vi "Script Tester.vi"() -> ()   [LabVIEW 2014]
panel:
  out "IN":bool
  out "OUT":bool
  in  "Execution Speed":u32(slide) scale=0.0..2000.0
  out "Function Code":picture
  out "Function Icon":picture
  in  "Evaluate":bool
  in  "OK":bool
  out "Status Msg":string
  out "Script":string
  in  "Test Script Path":path
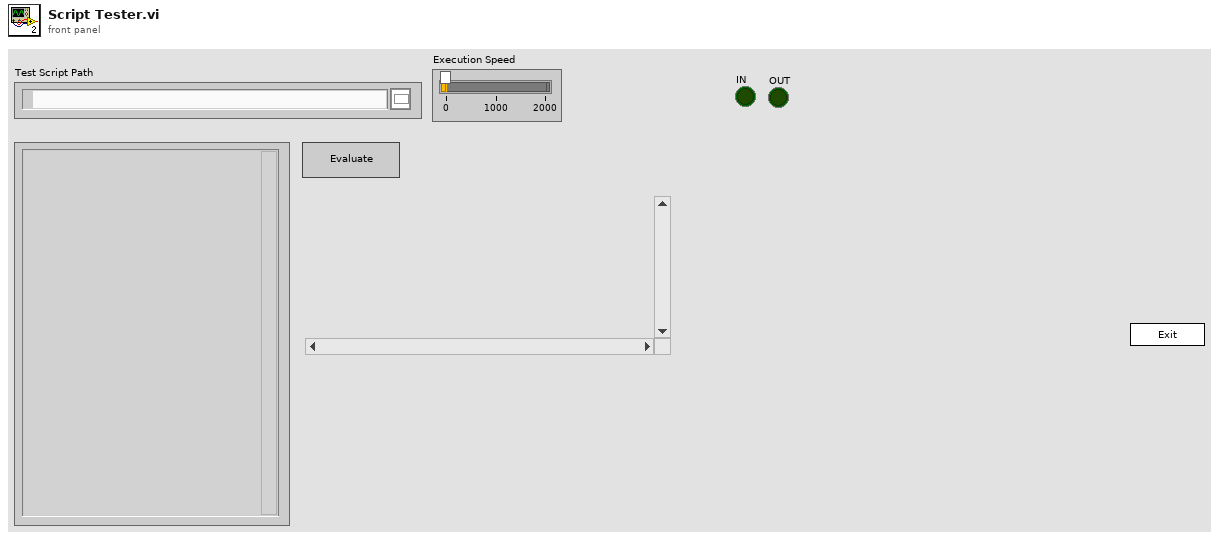
[diagram p1: front panel]
types:
  T1 = enum32{"invalid app kind", "Development System", "Run Time System", "Student Edition", "Embedded LabVIEW", "Evaluation", "Custom"}
  T2 = enum32{"Invalid", "Standard", "Closed", "Hidden", "Minimized", "Maximized"}
  T3 = enum32{"Bad", "Idle", "Run top level", "Running"}
  T4 = cluster{"Core":cluster{"Current VI Reference":refnum<vi>, "Close Panel on Exit?":bool}, "Test Script Path":path, "Script":string, "Function Path":path, "Script Pins":string[], "Function Pins":string[], "Function VI Ref":refnum<vi>}
  T5 = cluster{"Current VI Reference":refnum<vi>, "Close Panel on Exit?":bool}
  T6 = typedef "imagedata.ctl" = cluster{"image type":i32, "image depth":i32, "image":u8[], "mask":u8[], "colors":u32[], "Rectangle":cluster{"left":i16, "top":i16, "right":i16, "bottom":i16}}
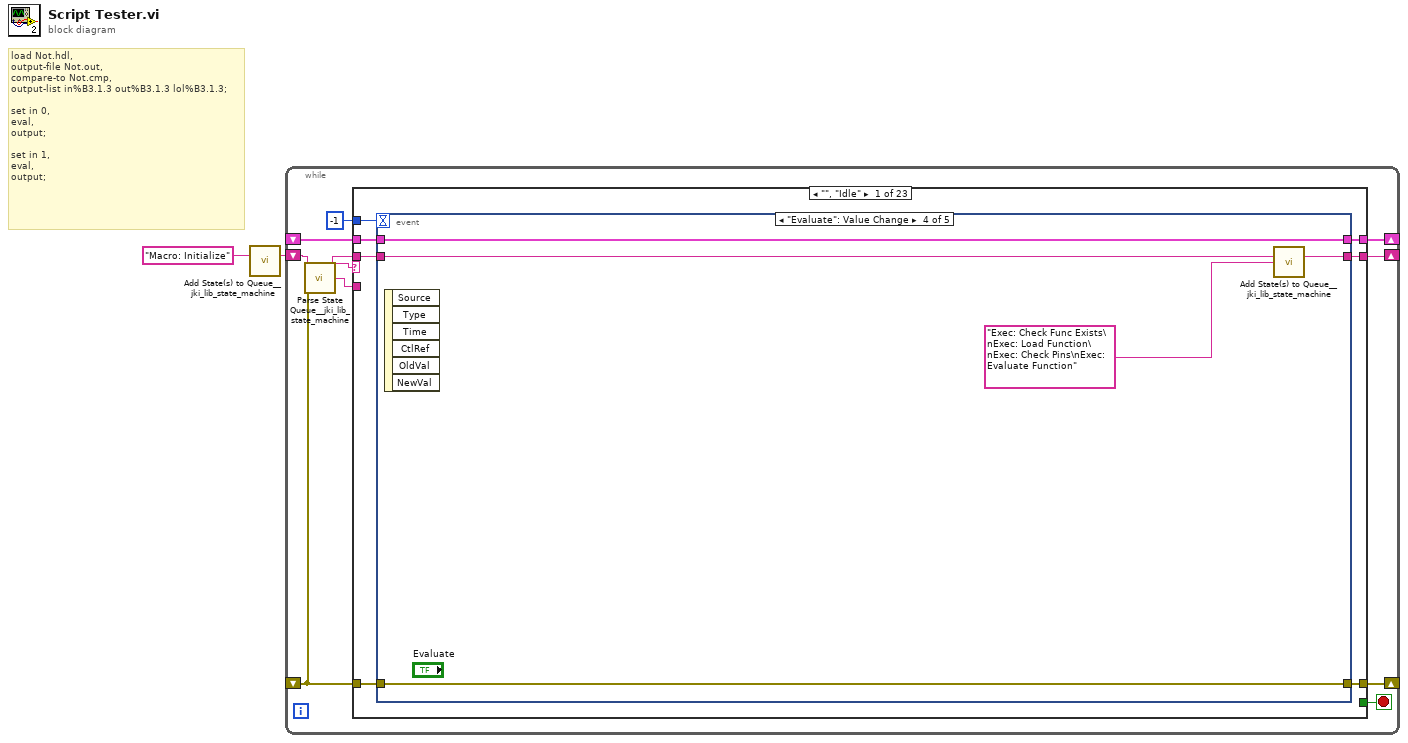
[diagram p0: block diagram]
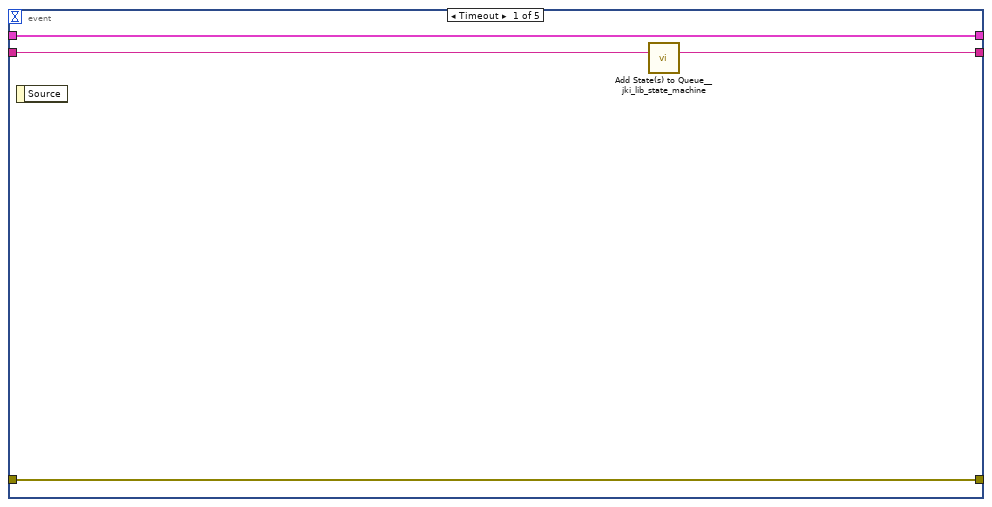
[diagram p2: hidden frame]
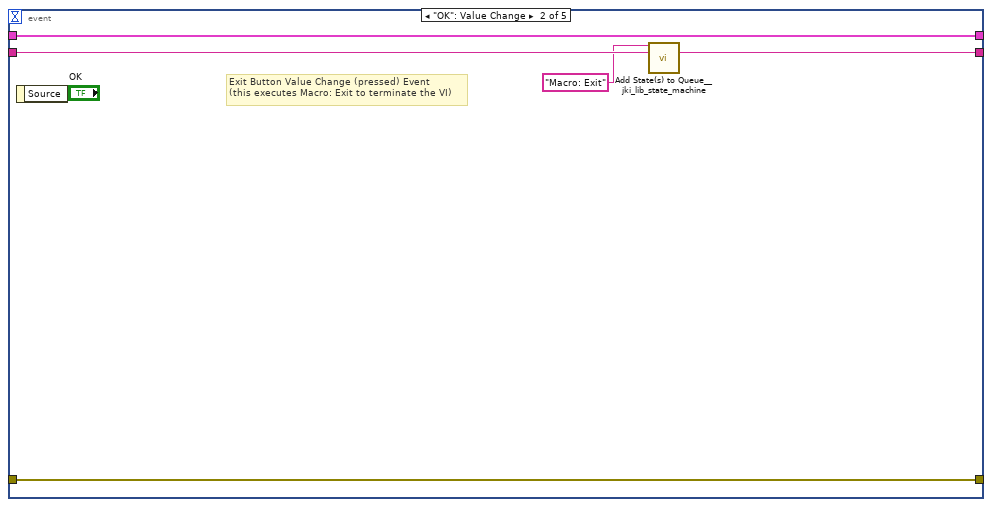
[diagram p3: hidden frame]
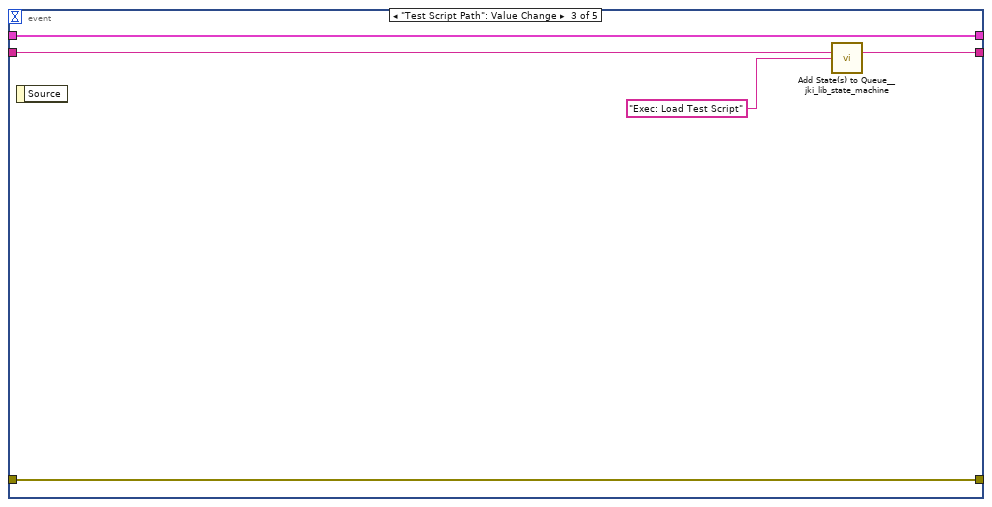
[diagram p4: hidden frame]
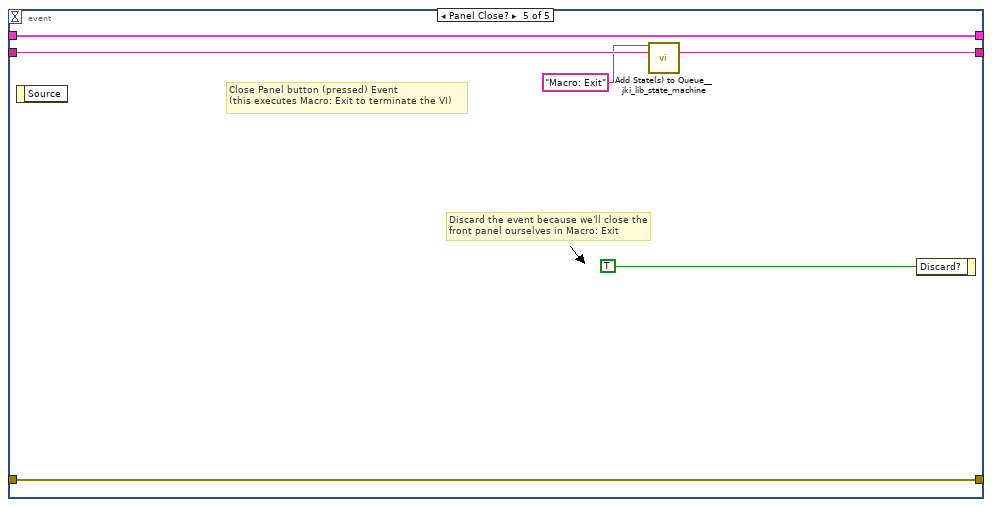
[diagram p5: hidden frame]
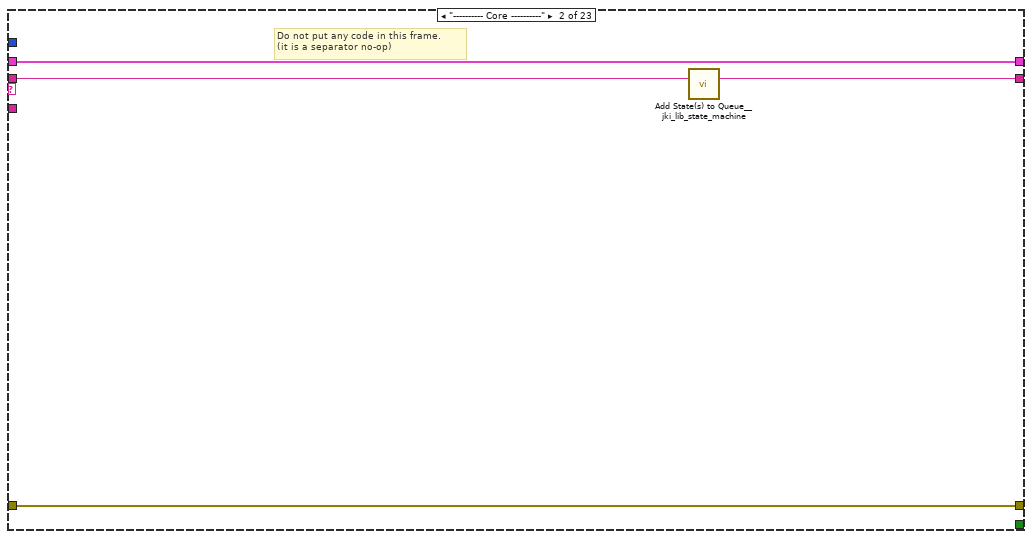
[diagram p6: hidden frame]
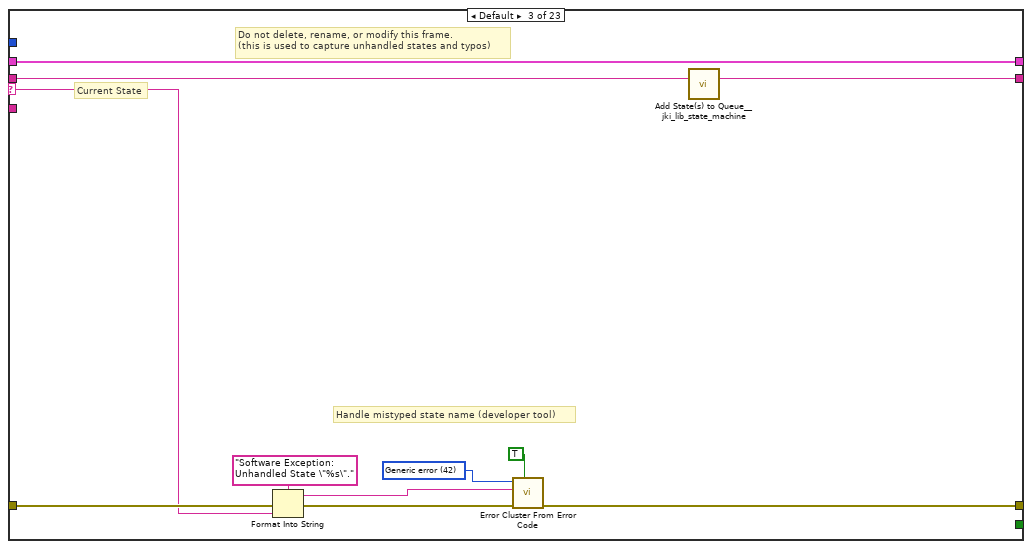
[diagram p7: hidden frame]
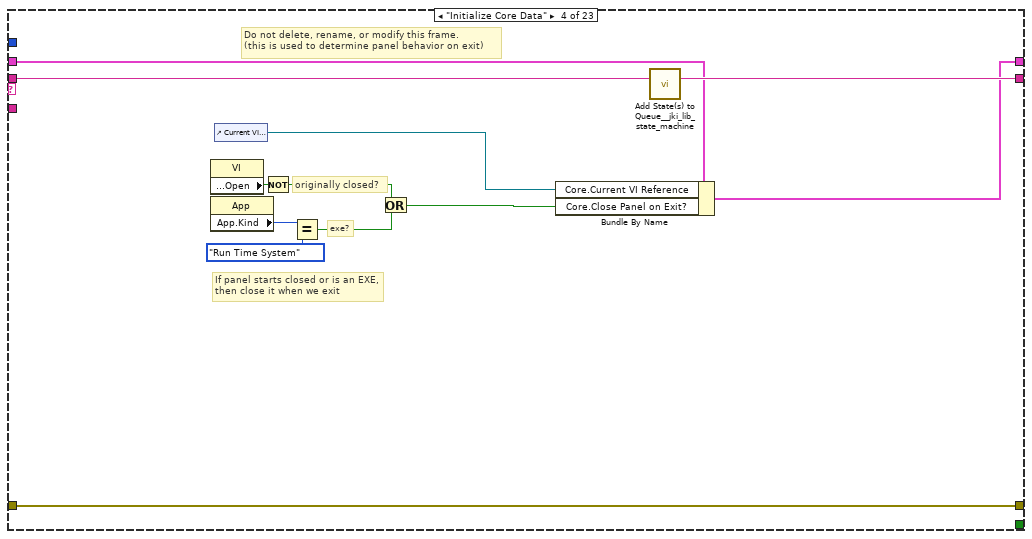
[diagram p8: hidden frame]
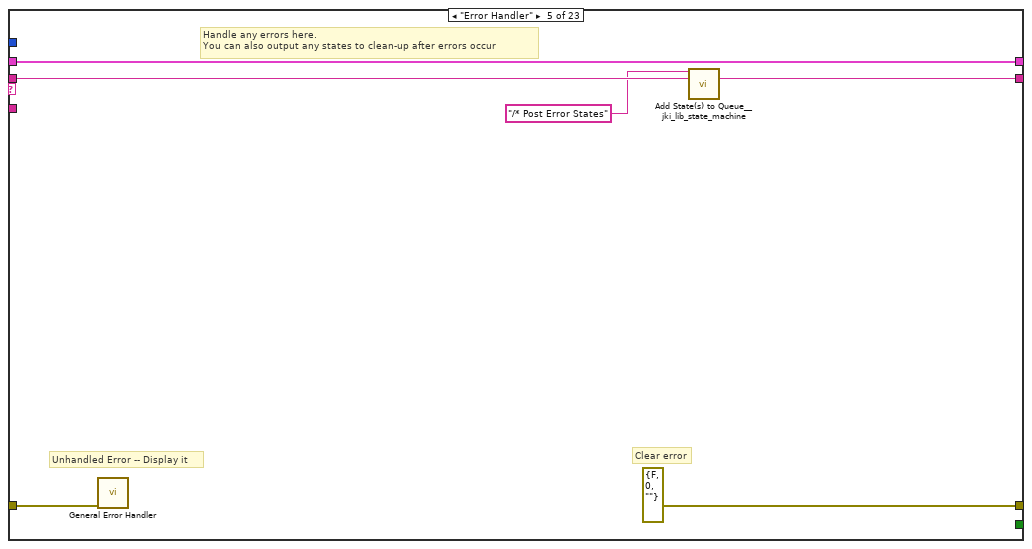
[diagram p9: hidden frame]
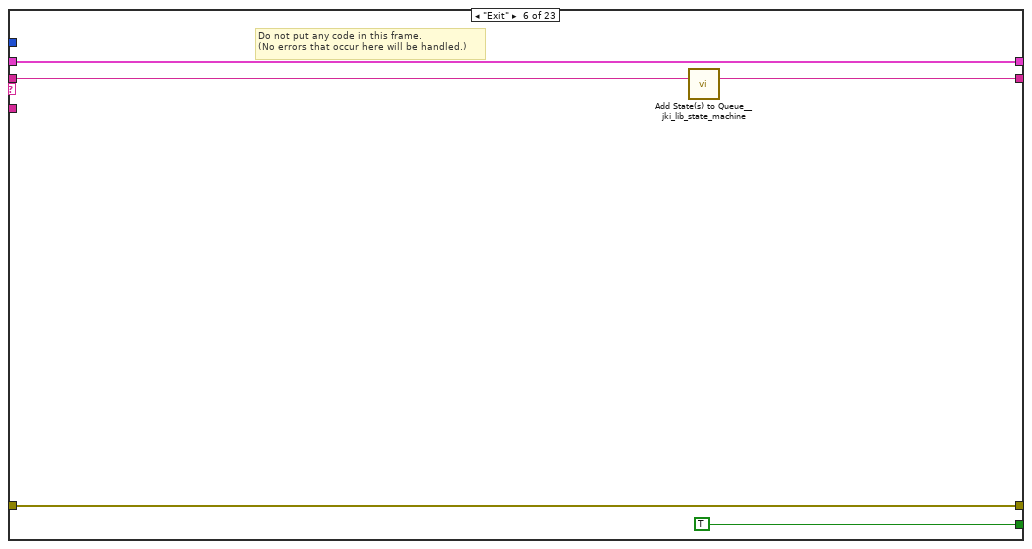
[diagram p10: hidden frame]
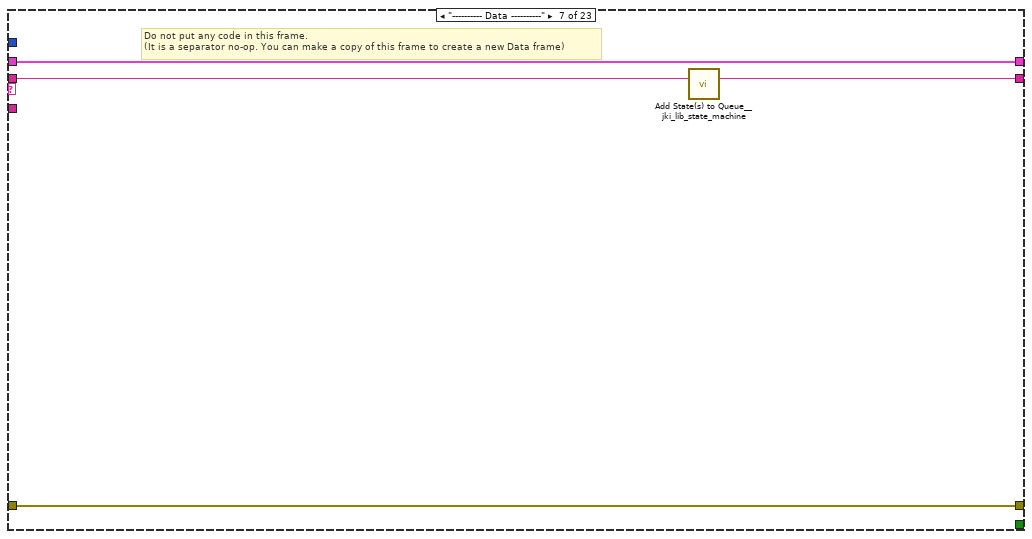
[diagram p11: hidden frame]
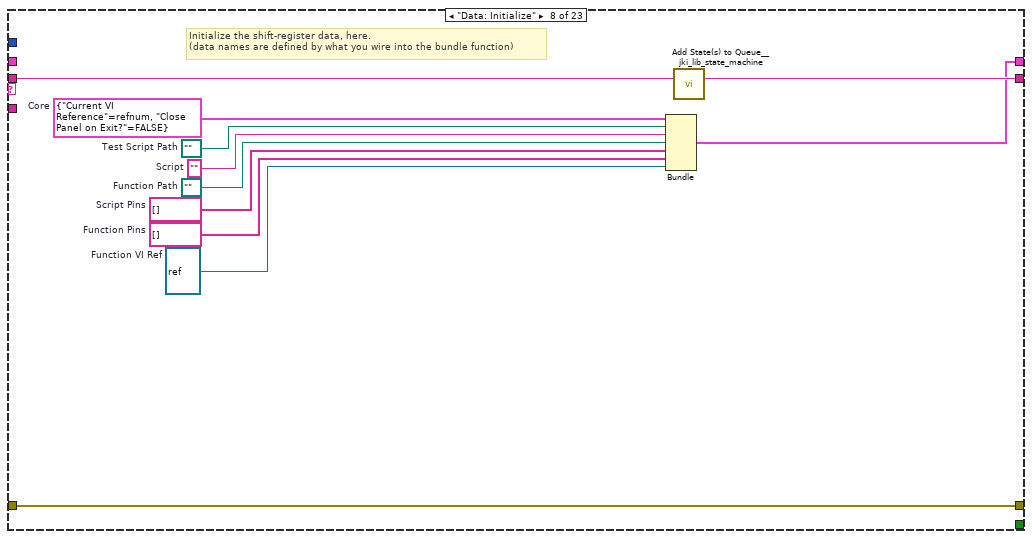
[diagram p12: hidden frame]
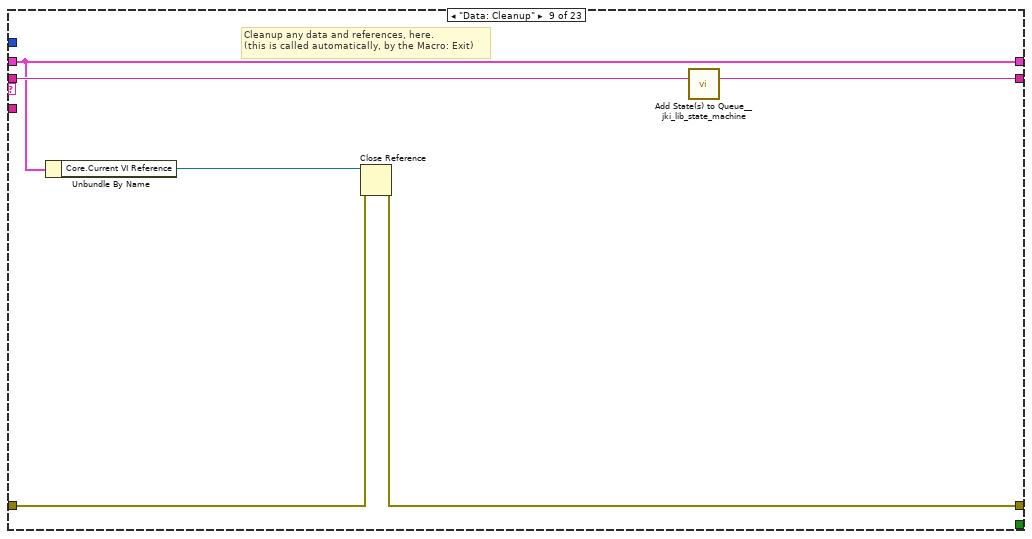
[diagram p13: hidden frame]
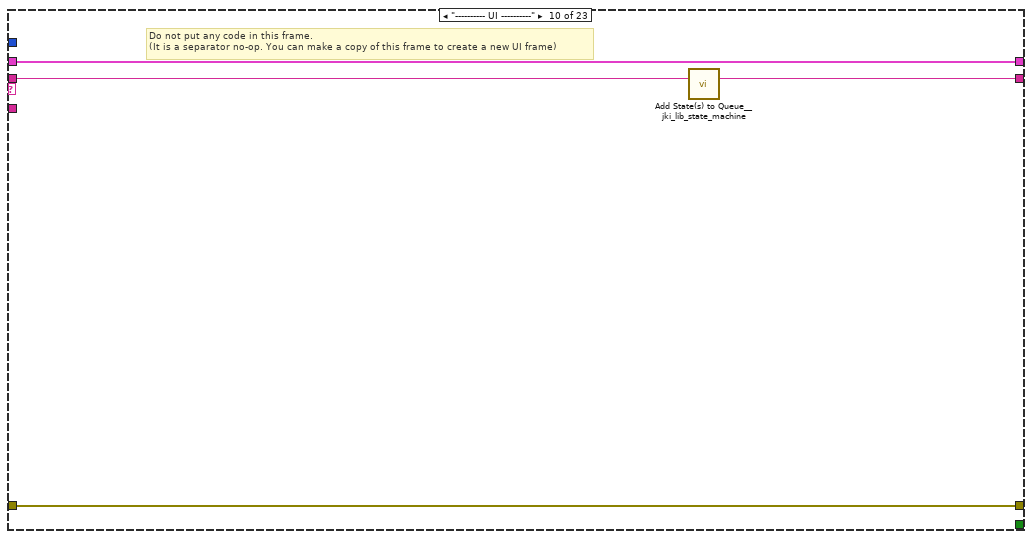
[diagram p14: hidden frame]
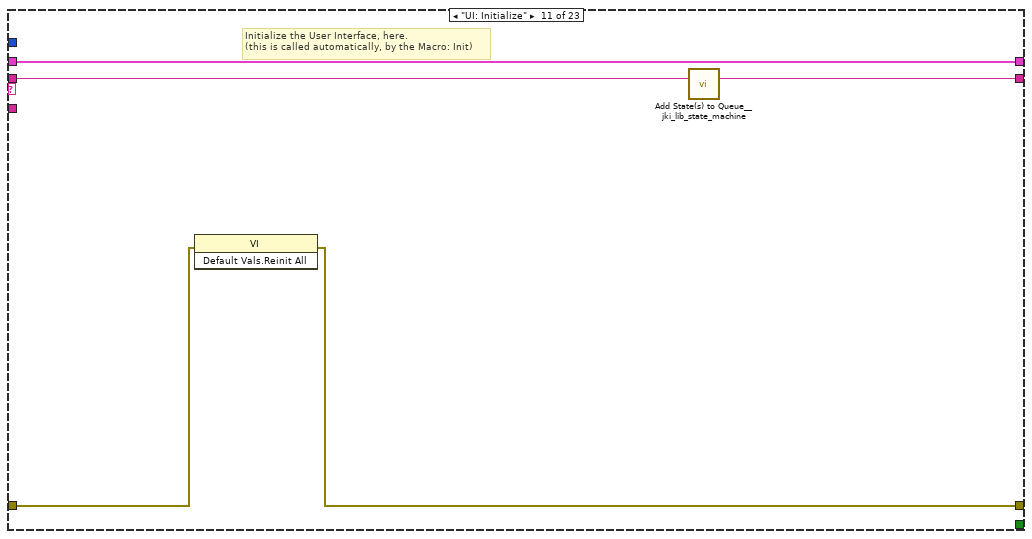
[diagram p15: hidden frame]
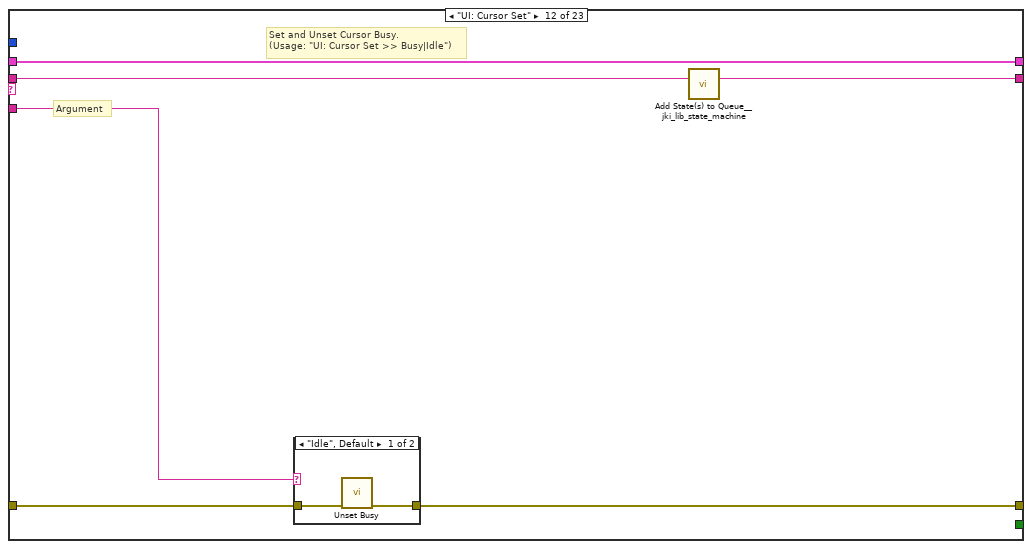
[diagram p16: hidden frame]
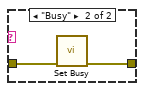
[diagram p17: hidden frame]
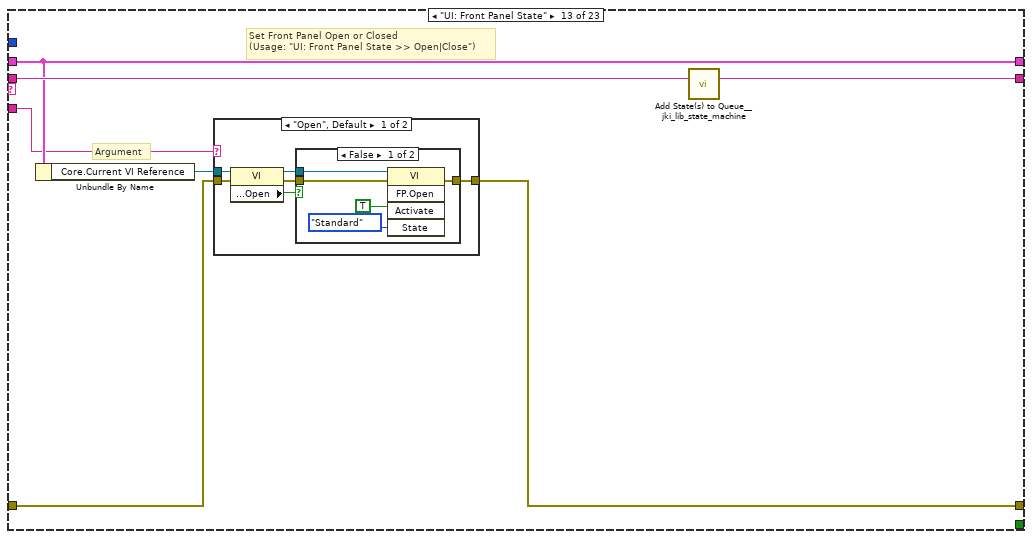
[diagram p18: hidden frame]
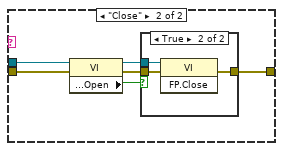
[diagram p20: hidden frame]
diagram:
  # "load Not.hdl,\noutput-file Not.out,\ncompare-to Not.cmp,\noutput-list in%B3.1.3 out%B3.1.3 lol%B3.1.3;\n\nset in 0,\neval,\noutput;\n\nset in 1,\neval,\noutput;"
  n1 = call <vilib>:"Add State(s) to Queue__jki_lib_state_machine.vi"("State(s) in (\"\")"="Macro: Initialize") -> ("States Out"=w2:string)  [unwired: 14 in]
  n2 = while {
    shift-right: [w6] -> _
    shift-left: _ -> [w5]
    shift-right: [w9] -> _
    shift-left: _ -> [w3]
    shift-right: [w8] -> _
    shift-left: w2 -> [w10]
    stop <- w7 stop-if-true
    n3 = call <vilib>:"Parse State Queue__jki_lib_state_machine.vi"("State Queue"=w10, "Error In (no error)"=w3) -> ("Remaining States"=w12:string, "Current State"=w13:string, "Arguments"=w11:string)  [unwired: 11 in]
    n4 = case shown="\"\", \"Idle\"" w13 {
      selector: w13 -> [_ _ w50 _ _ _ _ _ _ _ _ _ _ _ _ _ _ _ _ _ _ _ _]
      tunnel: w12 -> [w20 w49 w54 w72 w78 w83 w87 w98 w104 w108 w113 w119 w130 w157 w161 w166 w176 w180 w186 w235 w245 w286 _]
      tunnel: w11 -> [_ _ _ _ _ _ _ _ _ _ _ w114 w124 w153 _ _ _ _ _ _ _ _ _]
      tunnel: w5 -> [w18 w46 w52 w63 w75 w81 w84 _ w99 w105 w111 w117 w126 w155 w158 w163 w173 w177 w188 w223 w259 w295 w305]
      tunnel: [w17 w47 w56 w69 errorcluster {"status"=FALSE, "code"=0, "source"=""} ("error out") w80 w85 w95 w100 w106 w109 w115 w127 w154 w159 w164 w174 w178 w183 w237 w248 w294 w301] -> w9
      tunnel: w3 -> [w16 w47 w55 w69 w74 w80 w85 w95 w101 w106 w110 w116 w128 w154 w159 w164 w174 w178 w184 w238 w257 w294 w302]
      tunnel: [w19 w48 w53 w71 w77 w82 w86 w97 w103 w107 w112 w118 w129 w156 w160 w165 w175 w179 w191 w240 w260 w296 w306] -> w8
      tunnel: [_ _ _ _ _ TRUE _ _ _ _ _ _ _ _ _ _ _ _ _ _ _ _ _] -> w7
      tunnel: [w15 w46 w52 w70 w75 w81 w84 w96 w99 w105 w111 w117 w126 w155 w158 w163 w173 w177 w187 w222 w258 w295 w305] -> w6
      tunnel: -1 -> [w14 _ _ _ _ _ _ _ _ _ _ _ _ _ _ _ _ _ _ _ _ _ _]
      frame "", "Idle" {
        n5 = event shown="[3] \"Evaluate\": Value Change" {
          selector: _ -> [_ _ _ _ _]
          dyn-events: _ -> [_ _ _ _ _]
          timeout: w14 -> [_ _ _ _ _]
          tunnel: w20 -> [w24 w29 w33 w36 w45]
          tunnel: [w23 w28 w34 w37 w44] -> w19
          tunnel: w18 -> [w21 w26 w32 w38 w42]
          tunnel: [w22 w27 w30 w39 w43] -> w17
          tunnel: w16 -> [w22 w27 w30 w39 w43]
          tunnel: [w21 w26 w32 w38 w42] -> w15
          event Timeout {
            n6 = event-data() -> ()  [unwired: 1 in, 1 out]
            n7 = call <vilib>:"Add State(s) to Queue__jki_lib_state_machine.vi"("State(s) in (\"\")"=w24) -> ("States Out"=w23:string)  [unwired: 14 in]
          }
          event "OK": Value Change {
            # "Exit Button Value Change (pressed) Event\n(this executes Macro: Exit to terminate the VI)"
            n8 = event-data() -> ()  [unwired: 1 in, 1 out]
            n9 = call <vilib>:"Add State(s) to Queue__jki_lib_state_machine.vi"("State(s) in Front (\"\")"="Macro: Exit", "State(s) in (\"\")"=w29) -> ("States Out"=w28:string)  [unwired: 13 in]
          }
          event "Test Script Path": Value Change {
            n10 = event-data() -> ()  [unwired: 1 in, 1 out]
            n11 = call <vilib>:"Add State(s) to Queue__jki_lib_state_machine.vi"("State(s) in (\"\")"=w33, "State(s) at Back (\"\")"="Exec: Load Test Script" ("State(s) at Back (\"\")")) -> ("States Out"=w34:string)  [unwired: 13 in]
          }
          event "Evaluate": Value Change {
            n12 = event-data() -> ()  [unwired: 1 in, 6 out]
            n13 = call <vilib>:"Add State(s) to Queue__jki_lib_state_machine.vi"("State(s) in (\"\")"=w36, "State(s) at Back (\"\")"="Exec: Check Func Exists\nExec: Load Function\nExec: Check Pins\nExec: Evaluate Function" ("State(s) at Back (\"\")")) -> ("States Out"=w37:string)  [unwired: 13 in]
          }
          event Panel Close? {
            # "Discard the event because we'll close the front panel ourselves in Macro: Exit"
            # "Close Panel button (pressed) Event\n(this executes Macro: Exit to terminate the VI)"
            n14 = event-data() -> ()  [unwired: 1 in, 1 out]
            n15 = call <vilib>:"Add State(s) to Queue__jki_lib_state_machine.vi"("State(s) in Front (\"\")"="Macro: Exit", "State(s) in (\"\")"=w45) -> ("States Out"=w44:string)  [unwired: 13 in]
            n16 = event-data("Discard?"=TRUE) -> ()  [unwired: 1 in, 1 out]
          }
        }
      }
      frame "---------- Core ----------" {
        # "Do not put any code in this frame.\n(it is a separator no-op)"
        n17 = call <vilib>:"Add State(s) to Queue__jki_lib_state_machine.vi"("State(s) in (\"\")"=w49) -> ("States Out"=w48:string)  [unwired: 14 in]
      }
      frame Default {
        w59 = 42 items=["No error", "Argument error", "Memory is full", "Out of zone", "End of file", "File already open", "Generic file I/O error", "File not found", "File permission error", "Disk is full", "Duplicate path", "Too many files open", "System feature not enabled", "Resource file not found", "Cannot add resource", "Resource not found", "Image not found", "Image memory error", "Pen does not exist", "Config type invalid", "Config token not found", "Config parse error", "Config memory error", "Bad external code format", "Bad external code offset", "External code not present", "Null window", "Destroy window error", "Null menu", "Print aborted", "Bad print record", "Print driver error", "Windows error during printing", "Memory error during printing", "Print dialog error", "Generic print error", "Invalid device refnum", "Device not found", "Device parameter error", "Device unit error", "Cannot open device", "Device call aborted", "Generic error", "Cancelled by user", "Object ID too low", "Object ID too high", "Object not in heap", "Unknown heap", "Unknown object (invalid DefProc)", "Unknown object (DefProc not in table)", "Message out of range", "Invalid (null) method", "Unknown message", "Manager call not supported", "Bad address", "Network operation in progress", "Network operation timed out", "Connection is busy", "Network attribute not supported", "Network error", "Address in use", "System out of memory", "Connection aborted", "Connection refused", "Not connected", "Already connected", "Connection closed", "Initialization error (interapplication manager)", "Bad occurrence", "Wait on unbound occurrence handler", "Occurrence queue overflow", "Datalog type conflict", "Unused", "Unrecognized type (interapplication manager)", "Memory corrupt", "Failed to make temporary DLL", "Old CIN version", "Drag socket not found", "Failed to load drop-object", "Failed to register OLE object", "Failed to release OLE object", "Format specifier type mismatch", "Unknown format specifier", "Too few format specifiers", "Too many format specifiers", "Scan failed", "Newer CIN version", "Error converting to variant", "Runtime menu error", "Password tampered", "Variant attribute not found", "Incompatible variant data type", "Event data is not available", "Event Store is not present", "Occurrence is not found", "Event Queue is not created", "Event info is not available", "Refnum passed is NULL", "Error retrieving Class GUID", "Error retrieving CoClass GUID", "Error retrieving TypeLib GUID.", "Bad built application magic bytes.", "Specific driver is different from the specific driver associated with the Logical Name.", "There is no session opened to the class driver.", "Max Error", "MAX - Error with config objects", "MAX - Error loading configuration", "MAX - Group not supported"]
        # "Current State"
        # "Do not delete, rename, or modify this frame.\n(this is used to capture unhandled states and typos)"
        # "Handle mistyped state name (developer tool)"
        n18 = Format Into String(format string="Software Exception: Unhandled State \"%s\"." ("message"), error in=w55, w50) -> (resulting string=w58:string, error out=w57:errorcluster)  [unwired: 1 in]
        n19 = call <vilib>:"Error Cluster From Error Code.vi"("show call chain? (False)"=TRUE, "error in (no error)"=w57, "error message (\"\")"=w58, "error code (0)"=w59) -> ("error out"=w56:errorcluster)  [unwired: 5 in]
        n20 = call <vilib>:"Add State(s) to Queue__jki_lib_state_machine.vi"("State(s) in (\"\")"=w54) -> ("States Out"=w53:string)  [unwired: 14 in]
      }
      frame "Initialize Core Data" {
        # "Do not delete, rename, or modify this frame.\n(this is used to determine panel behavior on exit)"
        # "originally closed?"
        # "exe?"
        # "If panel starts closed or is an EXE, then close it when we exit"
        n21 = property class="VI"() -> ("Front Panel.Open"=w68:bool)  [unwired: 2 in, 2 out]
        n22 = property class="App"() -> ("App.Kind"=w67:T1)  [unwired: 2 in, 2 out]
        n23 = control-ref of="Current VI Reference"() -> (w61:refnum<vi>)
        n24 = Not(x=w68) -> (.not. x?=w65:bool)
        n25 = Equal?(x=w67, y=T1."Run Time System" ("Application:Kind")) -> (x = y?=w64:bool)
        n26 = Or(x=w65, y=w64) -> (x .or. y?=w62:bool)
        n27 = Bundle By Name(cluster=w63, "Core.Current VI Reference"=w61, "Core.Close Panel on Exit?"=w62) -> (w70:T4)
        n28 = call <vilib>:"Add State(s) to Queue__jki_lib_state_machine.vi"("State(s) in (\"\")"=w72) -> ("States Out"=w71:string)  [unwired: 14 in]
      }
      frame "Error Handler" {
        # "Unhandled Error -- Display it"
        # "Handle any errors here.\nYou can also output any states to clean-up after errors occur"
        # "Clear error"
        n29 = call <vilib>:"General Error Handler.vi"("error in (no error)"=w74) -> ()  [unwired: 10 in, 5 out]
        n30 = call <vilib>:"Add State(s) to Queue__jki_lib_state_machine.vi"("State(s) in Front (\"\")"="/* Post Error States", "State(s) in (\"\")"=w78) -> ("States Out"=w77:string)  [unwired: 13 in]
      }
      frame "Exit" {
        # "Do not put any code in this frame.\n(No errors that occur here will be handled.)"
        n31 = call <vilib>:"Add State(s) to Queue__jki_lib_state_machine.vi"("State(s) in (\"\")"=w83) -> ("States Out"=w82:string)  [unwired: 14 in]
      }
      frame "---------- Data ----------" {
        # "Do not put any code in this frame.\n(It is a separator no-op. You can make a copy of this frame to create a new Data frame)"
        n32 = call <vilib>:"Add State(s) to Queue__jki_lib_state_machine.vi"("State(s) in (\"\")"=w87) -> ("States Out"=w86:string)  [unwired: 14 in]
      }
      frame "Data: Initialize" {
        w88 = refnum<vi> refnum  # Function VI Ref
        w89 = string[] []  # Function Pins
        w90 = string[] []  # Script Pins
        w91 = path ""  # Function Path
        w92 = ""  # Script
        w93 = path ""  # Test Script Path
        w94 = T5 {"Current VI Reference"=refnum, "Close Panel on Exit?"=FALSE}  # Core
        # "Initialize the shift-register data, here.\n(data names are defined by what you wire into the bundle function)"
        n33 = Bundle("Core"=w94, "Test Script Path"=w93, "Script"=w92, "Function Path"=w91, "Script Pins"=w90, "Function Pins"=w89, "Function VI Ref"=w88) -> (w96:T4)  [unwired: 1 in]
        n34 = call <vilib>:"Add State(s) to Queue__jki_lib_state_machine.vi"("State(s) in (\"\")"=w98) -> ("States Out"=w97:string)  [unwired: 14 in]
      }
      frame "Data: Cleanup" {
        # "Cleanup any data and references, here.\n(this is called automatically, by the Macro: Exit)"
        n35 = Unbundle By Name(w99) -> ("Core.Current VI Reference"=w102:refnum<vi>)
        n36 = Close Reference(reference=w102, error in (no error)=w101) -> (error out=w100:errorcluster)
        n37 = call <vilib>:"Add State(s) to Queue__jki_lib_state_machine.vi"("State(s) in (\"\")"=w104) -> ("States Out"=w103:string)  [unwired: 14 in]
      }
      frame "---------- UI ----------" {
        # "Do not put any code in this frame.\n(It is a separator no-op. You can make a copy of this frame to create a new UI frame)"
        n38 = call <vilib>:"Add State(s) to Queue__jki_lib_state_machine.vi"("State(s) in (\"\")"=w108) -> ("States Out"=w107:string)  [unwired: 14 in]
      }
      frame "UI: Initialize" {
        # "Initialize the User Interface, here.\n(this is called automatically, by the Macro: Init)"
        n39 = invoke class="VI" method="Default Vals.Reinit All"(error in=w110) -> (error out=w109:errorcluster)  [unwired: 2 in, 2 out]
        n40 = call <vilib>:"Add State(s) to Queue__jki_lib_state_machine.vi"("State(s) in (\"\")"=w113) -> ("States Out"=w112:string)  [unwired: 14 in]
      }
      frame "UI: Cursor Set" {
        # "Argument"
        # "Set and Unset Cursor Busy.\n(Usage: \"UI: Cursor Set >> Busy|Idle\")"
        n41 = case shown="\"Idle\", Default" w114 {
          tunnel: w116 -> [w121 w123]
          tunnel: [w120 w122] -> w115
          frame "Idle", Default {
            n42 = call <vilib>:"Unset Busy.vi"("error in (no error)"=w121) -> ("error out"=w120:errorcluster)  [unwired: 10 in]
          }
          frame "Busy" {
            n43 = call <vilib>:"Set Busy.vi"("error in (no error)"=w123) -> ("error out"=w122:errorcluster)  [unwired: 9 in, 1 out]
          }
        }
        n44 = call <vilib>:"Add State(s) to Queue__jki_lib_state_machine.vi"("State(s) in (\"\")"=w119) -> ("States Out"=w118:string)  [unwired: 14 in]
      }
      frame "UI: Front Panel State" {
        # "Argument"
        # "Set Front Panel Open or Closed\n(Usage: \"UI: Front Panel State >> Open|Close\")"
        n45 = Unbundle By Name(w126) -> ("Core.Current VI Reference"=w125:refnum<vi>)
        n46 = case shown="\"Open\", Default" w124 {
          tunnel: w128 -> [w134 w147]
          tunnel: [w136 w148] -> w127
          tunnel: w125 -> [w135 w145]
          frame "Open", Default {
            n47 = property class="VI"(reference=w135, error in=w134) -> (reference out=w132:refnum<vi>, error out=w133:errorcluster, "Front Panel.Open"=w131:bool)
            n48 = case shown="False" w131 {
              tunnel: [w139 w142] -> w136
              tunnel: w133 -> [w138 w142]
              tunnel: w132 -> [w137 _]
              frame False {
                n49 = invoke class="VI" method="FP.Open"(reference=w137, error in=w138, "Activate"=TRUE, "State"=T2."Standard") -> (error out=w139:errorcluster)  [unwired: 1 in, 4 out]
              }
              frame True {
              }
            }
          }
          frame "Close" {
            n50 = property class="VI"(reference=w145, error in=w147) -> (reference out=w144:refnum<vi>, error out=w146:errorcluster, "Front Panel.Open"=w143:bool)
            n51 = case shown="True" w143 {
              tunnel: [w149 w152] -> w148
              tunnel: w146 -> [w149 w151]
              tunnel: w144 -> [_ w150]
              frame False {
              }
              frame True {
                n52 = invoke class="VI" method="FP.Close"(reference=w150, error in=w151) -> (error out=w152:errorcluster)  [unwired: 1 in, 2 out]
              }
            }
          }
        }
        n53 = call <vilib>:"Add State(s) to Queue__jki_lib_state_machine.vi"("State(s) in (\"\")"=w130) -> ("States Out"=w129:string)  [unwired: 14 in]
      }
      frame "UI: Set Status Msg" {
        # "Set Status Msg\n(Usage: \"UI: Set Status Msg >> Message\")"
        n54 = call <vilib>:"Add State(s) to Queue__jki_lib_state_machine.vi"("State(s) in (\"\")"=w157) -> ("States Out"=w156:string)  [unwired: 14 in]
        "Status Msg" <- w153
      }
      frame "---------- Macro ----------" {
        # "Do not put any code in this frame.\n(It is a separator no-op. You can make a copy of this frame to create a new Macro frame)"
        n55 = call <vilib>:"Add State(s) to Queue__jki_lib_state_machine.vi"("State(s) in (\"\")"=w161) -> ("States Out"=w160:string)  [unwired: 14 in]
      }
      frame "Macro: Initialize" {
        w162 = "Data: Initialize\nInitialize Core Data\nUI: Initialize\nUI: Front Panel State >> Open"  # Data: Initialize Initialize Core Data UI: Initialize UI: Front Panel State >> Open
        # "Initialization Macro\n(This is called once, when the VI starts)"
        n56 = call <vilib>:"Add State(s) to Queue__jki_lib_state_machine.vi"("State(s) in Front (\"\")"=w162, "State(s) in (\"\")"=w166) -> ("States Out"=w165:string)  [unwired: 13 in]
      }
      frame "Macro: Exit" {
        # "Exit Macro\n(This is called once, when the VI exits)"
        n57 = Unbundle By Name(w173) -> ("Core.Close Panel on Exit?"=w172:bool)
        n58 = Select(t="UI: Front Panel State >> Close", s=w172, f="") -> (s? t:f=w169:string)
        n59 = call <vilib>:"Add State(s) to Queue__jki_lib_state_machine.vi"("State(s) in (\"\")"=w169, "State(s) at Back (\"\")"="Data: Cleanup\nExit") -> ("States Out"=w167:string)  [unwired: 13 in]
        n60 = call <vilib>:"Add State(s) to Queue__jki_lib_state_machine.vi"("State(s) in Front (\"\")"=w167, "State(s) in (\"\")"=w176) -> ("States Out"=w175:string)  [unwired: 13 in]
      }
      frame "---------- Exec ----------" {
        # "Template Separator\n(You can make a copy of, or modify, this frame)"
        n61 = call <vilib>:"Add State(s) to Queue__jki_lib_state_machine.vi"("State(s) in (\"\")"=w180) -> ("States Out"=w179:string)  [unwired: 14 in]
      }
      frame "Exec: Load Test Script" {
        # "Loads Test Script"
        n62 = Empty String/Path?(string/path="Test Script Path") -> (empty?=w190:bool)
        n63 = case shown="False" w190 {
          tunnel: "Test Script Path" -> [w210 _]
          tunnel: w184 -> [w202 w220]
          tunnel: [w201 w220] -> w183
          tunnel: [w200 "UI: Set Status Msg >> Script Loading Cancelled by User"] -> w185
          tunnel: [w195 _] -> w182
          tunnel: [w192 _] -> w181
          frame False {
            n64 = Open/Create/Replace File(file path (use dialog)=w210, error in=w202) -> (refnum out=w208:refnum<file>, error out=w209:errorcluster)  [unwired: 4 in, 1 out]
            n65 = Read from Text File(file (use dialog)=w208, error in=w209) -> (refnum out=w207:refnum<file>, text=w195:string, error out=w206:errorcluster)  [unwired: 2 in, 1 out]
            n66 = Close File(refnum=w207, error in=w206) -> (path=w205:path, error out=w201:errorcluster)
            n67 = Path To String(path=w205) -> (string=w204:string)
            n68 = Concatenate Strings("UI: Set Status Msg >> New Script Loaded: ", w204) -> (w200:string)
            n69 = Match Pattern(string=w195, regular expression="output-list ") -> (after substring=w198:string)  [unwired: 1 in, 3 out]
            n70 = Match Pattern(string=w198, regular expression=";") -> (before substring=w196:string)  [unwired: 1 in, 3 out]
            n71 = while {
              shift-right: [w211] -> _
              shift-left: w196 -> [w218]
              tunnel: [w213] -> w193 mode=indexing
              stop <- w215 stop-if-true
              n72 = Match Pattern(string=w218, regular expression="%") -> (before substring=w213:string, after substring=w212:string, offset past match=w216:i32)  [unwired: 1 in, 1 out]
              n73 = Less Than 0?(x=w216) -> (x < 0?=w215:bool)
              n74 = Match Pattern(string=w212, regular expression="\\s") -> (after substring=w211:string)  [unwired: 1 in, 3 out]
            }
            n75 = Delete From Array(array=w193, length=1) -> (array with subset deleted=w192:string[])  [unwired: 1 in, 1 out]
          }
          frame True {
          }
        }
        "Script" <- w182
        n76 = Bundle By Name(cluster=w188, "Test Script Path"="Test Script Path", "Script"=w182, "Script Pins"=w181) -> (w187:T4)
        n77 = call <vilib>:"Add State(s) to Queue__jki_lib_state_machine.vi"("State(s) in (\"\")"=w186, "State(s) at Back (\"\")"=w185) -> ("States Out"=w191:string)  [unwired: 13 in]
      }
      frame "Exec: Check Func Exists" {
        # "Check if Function Exists Prior to opening it"
        n78 = Unbundle By Name(w223) -> ("Test Script Path"=w233:path)
        n79 = Strip Path(path=w233) -> (stripped path=w232:path, name=w230:string)
        n80 = Match Pattern(string=w230, regular expression="[.]") -> (before substring=w228:string)  [unwired: 1 in, 3 out]
        n81 = Concatenate Strings(w228, ".vi" ("string")) -> (w231:string)
        n82 = Build Path(base path=w232, name or relative path=w231) -> (appended path=w221:path)
        n83 = call <vilib>:"Check if File or Folder Exists.vi"("error in (no error)"=w238, "path"=w221) -> ("error out"=w237:errorcluster, "file or folder exists?"=w236:bool)  [unwired: 7 in, 1 out]
        n84 = Path To String(path=w221) -> (string=w227:string)
        n85 = Concatenate Strings("UI: Set Status Msg >> Function " ("f"), w227, " not found." ("string")) -> (w224:string)
        n86 = Select(t=w235, s=w236, f=w224) -> (s? t:f=w234:string)
        n87 = Bundle By Name(cluster=w223, "Function Path"=w221) -> (w222:T4)
        n88 = call <vilib>:"Add State(s) to Queue__jki_lib_state_machine.vi"("State(s) in (\"\")"=w234) -> ("States Out"=w240:string)  [unwired: 14 in]
      }
      frame "Exec: Load Function" {
        # "Carrega Function"
        n89 = Unbundle By Name(w259) -> ("Function Path"=w243:path)
        n90 = Path To String(path=w243) -> (string=w242:string)
        n91 = Open VI Reference(vi path=w243, error in (no error)=w257) -> (vi reference=w250:refnum<vi>, error out=w256:errorcluster)  [unwired: 4 in]
        n92 = property class="VI"(reference=w250, error in=w256) -> (error out=w251:errorcluster, "Panel"=w252:refnum<vi>, "Exec.State"=w255:T3)  [unwired: 1 out]
        n93 = Equal?(x=w255, y=T3."Idle") -> (x = y?=w253:bool)
        n94 = case shown="True" w253 {
          tunnel: w252 -> [_ w280]
          tunnel: w251 -> [w264 w279]
          tunnel: w250 -> [_ w276]
          tunnel: [_ w274] -> w249
          tunnel: [w264 w267] -> w248
          tunnel: [_ w272] -> w247
          tunnel: [_ w268] -> w246
          tunnel: w245 -> [_ w266]
          tunnel: [w261 w266] -> w244
          tunnel: w242 -> [w262 _]
          tunnel: [_ w265] -> w241
          frame False {
            # "Unusable State"
            n95 = Concatenate Strings("UI: Set Status Msg >> Function on an unknown state. Check " ("Remaining States"), w262) -> (w261:string)
          }
          frame True {
            # "VI Idle State"
            n96 = property class="Pnl"(reference=w280, error in=w279) -> (error out=w278:errorcluster, "Controls[]"=w277:refnum<vi>[])  [unwired: 1 out]
            n97 = for {
              tunnel: w277 -> [w283] mode=indexing
              tunnel: [w282] -> w274 mode=indexing
              shift-right: [w281] -> w275
              shift-left: w278 -> [w284]
              n98 = property class="Ctl"(reference=w283, error in=w284) -> (error out=w281:errorcluster, "Label.Text"=w282:string)  [unwired: 1 out]
            }
            n99 = invoke class="VI" method="VI Icon.Get as Image Data"(reference=w276, error in=w275) -> (reference out=w271:refnum<vi>, error out=w270:errorcluster, "ImageData"=w273:T6)  [unwired: 4 in, 3 out]
            n100 = call <vilib>:"Draw Flattened Pixmap.vi"("image data"=w273) -> ("new picture"=w272:picture)  [unwired: 8 in]
            n101 = invoke class="VI" method="BD.Get Image Scaled"(reference=w271, error in=w270) -> (reference out=w265:refnum<vi>, error out=w267:errorcluster, "img data"=w269:T6)  [unwired: 5 in, 4 out]
            n102 = call <vilib>:"Draw Flattened Pixmap.vi"("image data"=w269) -> ("new picture"=w268:picture)  [unwired: 8 in]
          }
        }
        "Function Icon" <- w247
        "Function Code" <- w246
        n103 = Bundle By Name(cluster=w259, "Function Pins"=w249, "Function VI Ref"=w241) -> (w258:T4)
        n104 = call <vilib>:"Add State(s) to Queue__jki_lib_state_machine.vi"("State(s) in (\"\")"=w244) -> ("States Out"=w260:string)  [unwired: 14 in]
      }
      frame "Exec: Check Pins" {
        # "Checks if Test Script and Function have the same pins"
        n105 = Unbundle By Name(w295) -> ("Function Pins"=w293:string[], "Script Pins"=w292:string[])
        n106 = for {
          tunnel: w293 -> [w300]
          tunnel: w292 -> [w297] mode=indexing
          tunnel: [w298] -> w291
          tunnel: [w297] -> w289
          stop <- w298 stop-if-true
          n107 = Search 1D Array(1D array=w300, element=w297) -> (index of element=w299:i32)  [unwired: 1 in]
          n108 = Less Than 0?(x=w299) -> (x < 0?=w298:bool)
        }
        n109 = Concatenate Strings("UI: Set Status Msg >> Pin ", w289, " not found on function" ("string")) -> (w287:string)
        n110 = Select(t=w287, s=w291, f=w286) -> (s? t:f=w285:string)
        n111 = call <vilib>:"Add State(s) to Queue__jki_lib_state_machine.vi"("State(s) in (\"\")"=w285) -> ("States Out"=w296:string)  [unwired: 14 in]
      }
      frame "Exec: Evaluate Function" {
        # "Evaluates Function According to Test Script"
        n112 = Unbundle By Name(w305) -> ("Function VI Ref"=w304:refnum<vi>, "Script"=w303:string)
        n113 = while {
          tunnel: w304 -> [w310]
          shift-right: [w307] -> _
          shift-left: w303 -> [w316]
          tunnel: w302 -> [w309]
          tunnel: [w308] -> w301
          stop <- w312 stop-if-true
          n114 = Match Pattern(string=w316, regular expression="set ") -> (after substring=w311:string, offset past match=w314:i32)  [unwired: 1 in, 2 out]
          n115 = Less Than 0?(x=w314) -> (x < 0?=w313:bool)
          n116 = case shown="False" w313 {
            tunnel: [_ TRUE] -> w312
            tunnel: w311 -> [w338 _]
            tunnel: w310 -> [w334 _]
            tunnel: w309 -> [w333 w339]
            tunnel: [w322 w339] -> w308
            tunnel: [w321 _] -> w307
            frame False {
              # "Test"
              n117 = Match Pattern(string=w338, regular expression="\\s") -> (before substring=w332:string, after substring=w336:string)  [unwired: 1 in, 2 out]
              n118 = Match Pattern(string=w336, regular expression=",") -> (before substring=w331:string, after substring=w321:string)  [unwired: 1 in, 2 out]
              n119 = Equal?(x=w331, y="1") -> (x = y?=w329:bool)
              "IN" <- w329
              n120 = invoke class="VI" method="Ctrl Val.Set"(reference=w334, error in=w333, "Control Name"=w332, "Value"=w329) -> (reference out=w320:refnum<vi>, error out=w328:errorcluster)  [unwired: 1 in, 3 out]
              n121 = invoke class="VI" method="Run VI"(reference=w320, "Wait until done"=TRUE ("Wait Until Done")) -> (reference out=w319:refnum<vi>)  [unwired: 3 in, 4 out]
              n122 = invoke class="VI" method="Ctrl Val.Get"(reference=w319, error in=w328, "Control Name"="out") -> (error out=w325:errorcluster, "Get Control Value Variant"=w326:variant)  [unwired: 1 in, 2 out]
              n123 = Variant To Data(error in=w325, type=TRUE, Variant=w326) -> (data=→"OUT":bool, error out=w322:errorcluster)
            }
            frame True {
              # "END"
            }
          }
          n124 = Wait (ms)(milliseconds to wait="Execution Speed") -> ()  [unwired: 1 out]
        }
        n125 = call <vilib>:"Add State(s) to Queue__jki_lib_state_machine.vi"() -> ("States Out"=w306:string)  [unwired: 15 in]
      }
    }
  }
